vi "Ball Collector SM 5.1.vi"(1 "FIRE":bool, 2 "REVERSE":bool, 3 "Intake Motor":bool, 4 "OVERRIDE":bool, 5 "OVERRIDE 2":bool, 8 "BB1":bool, 9 "1":bool, 10 "BB2":bool, 11 "2":bool, 12 "BB3":bool, 13 "3":bool, 14 "BB4":bool, 27 "new behavior":bool) -> (20 "Ball Count":dbl, 21 "Intake motor":dbl, 22 "Motor A 2":dbl, 23 "Motor B 3":dbl, 24 "Motor C":dbl)   [LabVIEW 2011]
panel:
  in  "Feed Delay (sec) 2":dbl=0.5
  in  "Feed Delay (sec)":dbl=0.5
  in  "Prime":dbl(knob)=0.20200759564815568 scale=0.0..1.0
  in  "FIRE":dbl(knob)=0.5049245430258039 scale=0.0..1.0
  out "C from 3":bool
  out "B from 2":bool
  out "A from 1":bool
  out "BSB State":enum16{"Ball Entered"}(ring)
  out "BSC":bool
  out "BSB":bool
  out "BSA":bool
  out "MC":enum16{"Stopped", "Foward", "Reverse"}(ring)
  out "MA":enum16{"Stopped", "Foward", "Reverse"}(ring)
  out "MB":enum16{"Stopped", "Foward", "Reverse"}(ring)
  out "Intake motor":bool
  out "C Status":string
  out "B Status":string
  out "A Status":string
  out "Ball System State":string
  out "Primed":bool
  out "MA":bool
  out "MB":bool
  out "MC":bool
  # "Upper System"
  # "Upper/Middle System (U/M)"
  # "Ball systems"
  # "Vacant = Black (T)\nOccupied = Orange (F)"
  # "Lower/Middle System (L/M)"
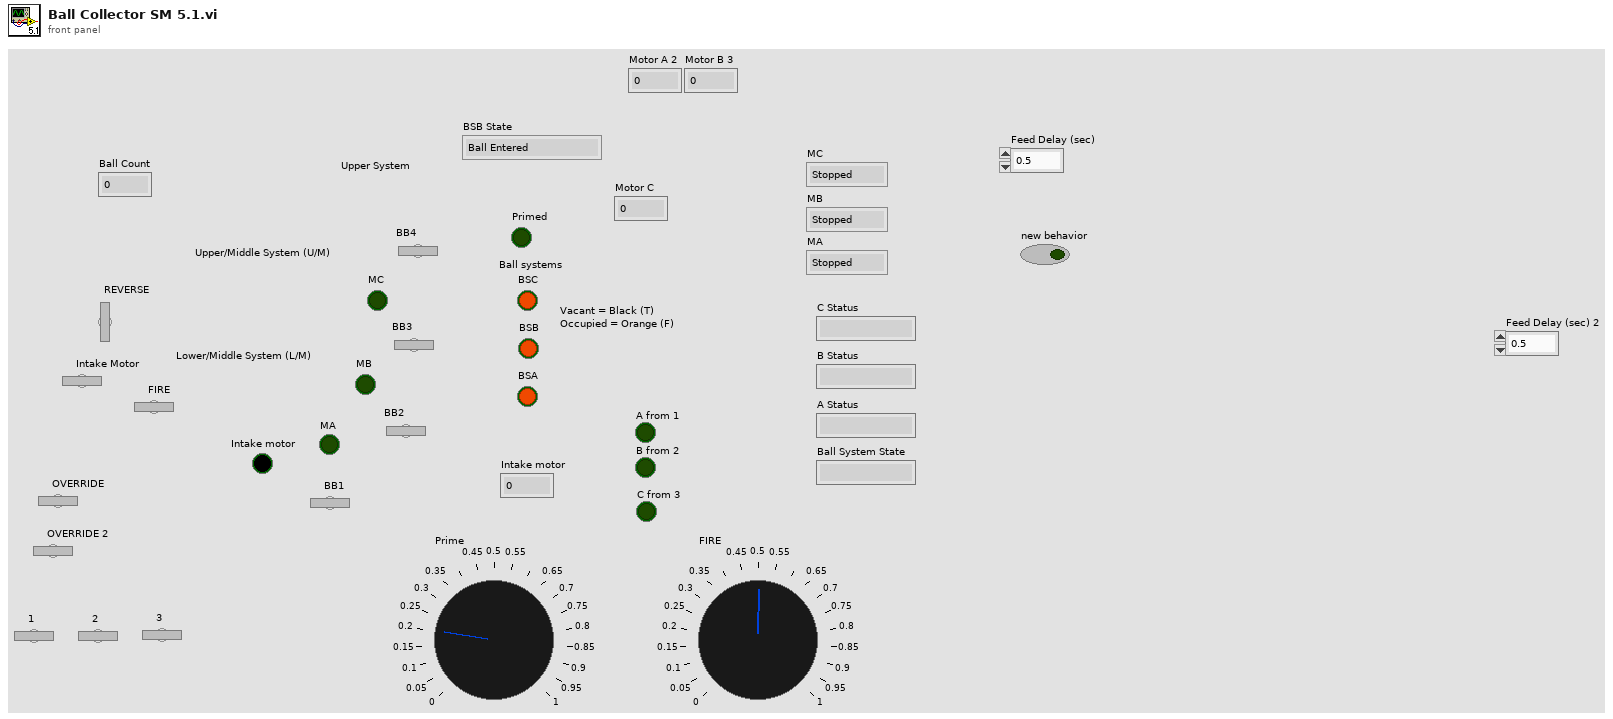
[diagram p1: front panel]
types:
  T1 = enum16{"Ball Entered", "Ball Stopped", "Ball Moveing", "Ball Leaving"}
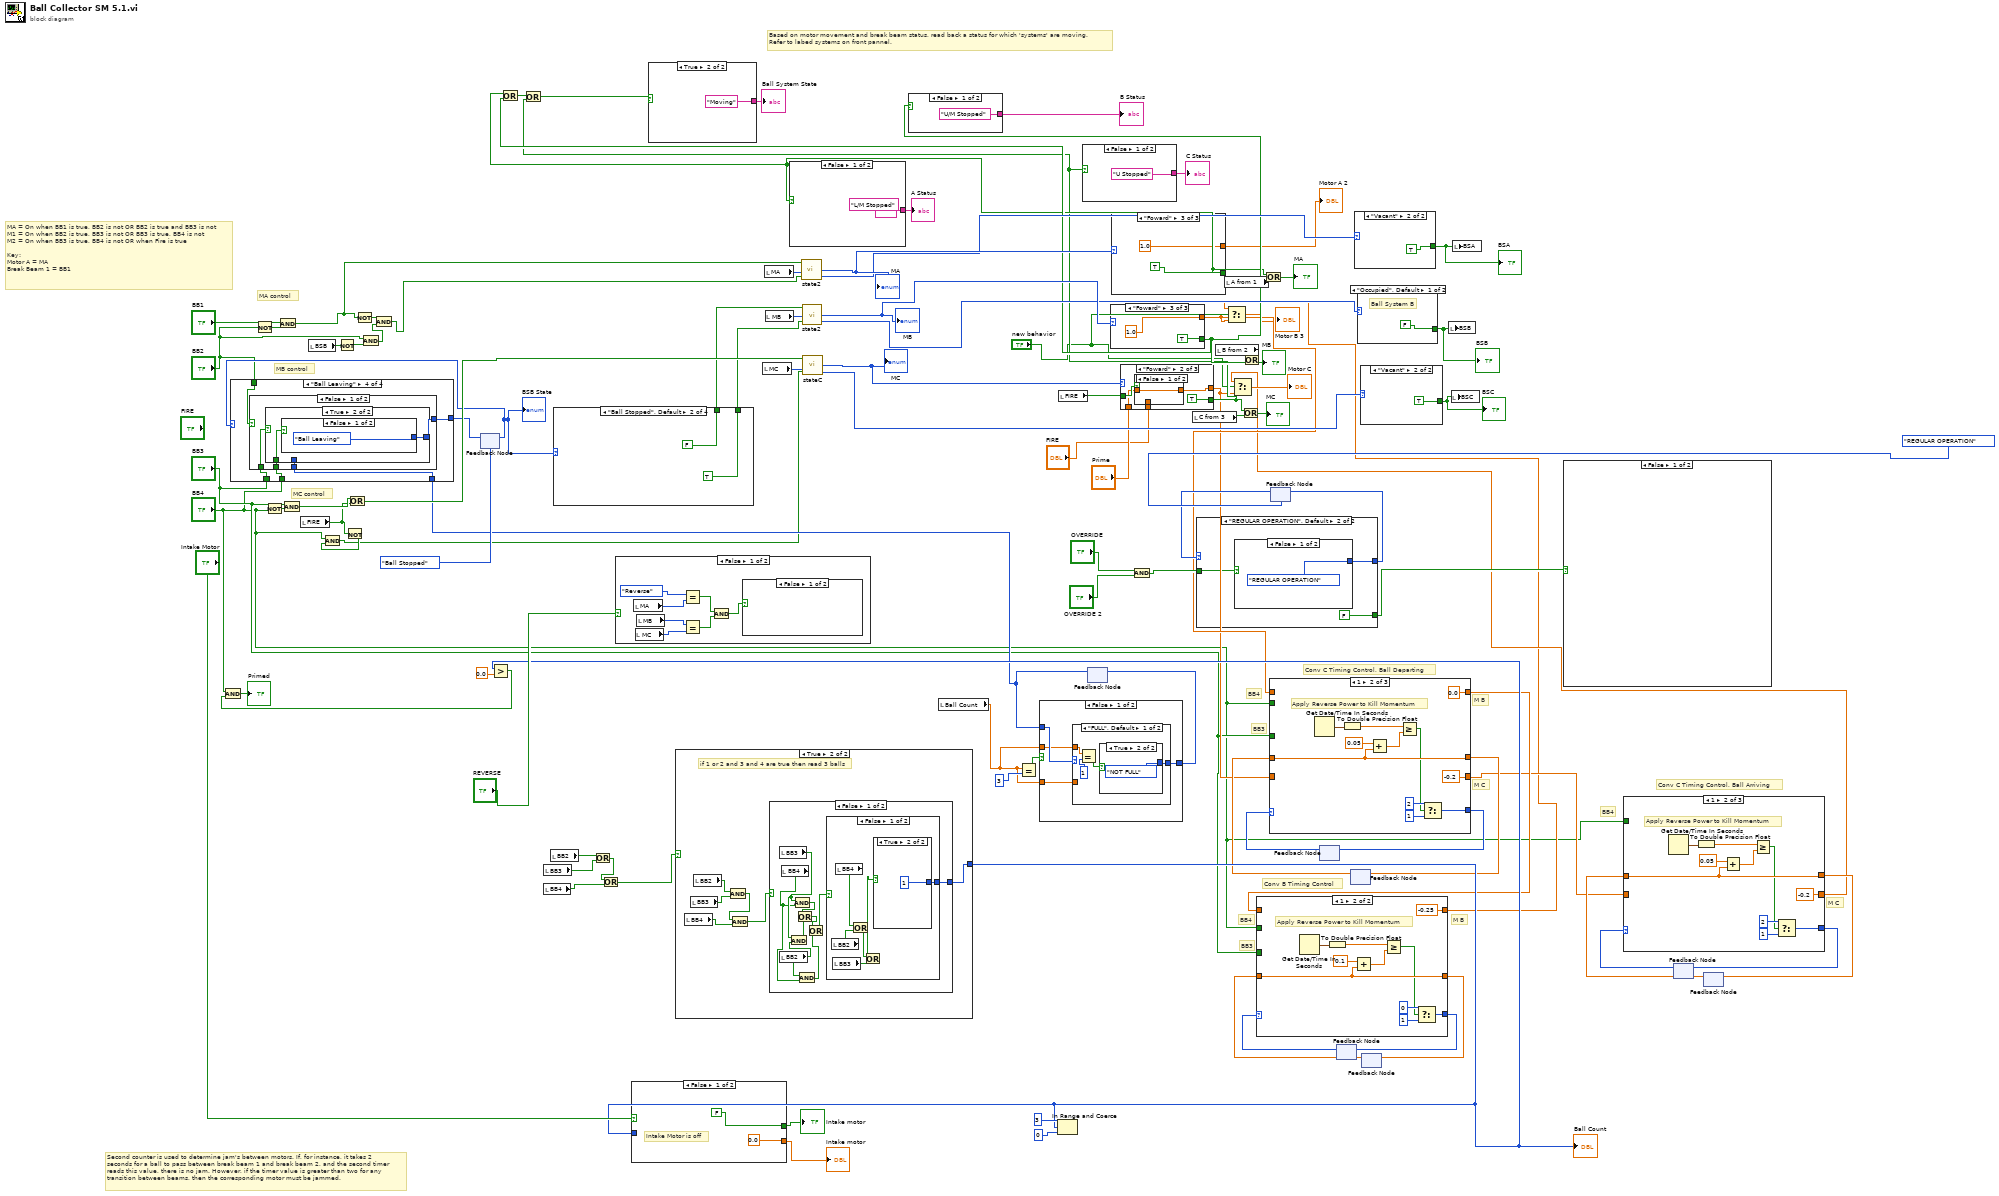
[diagram p0: block diagram]
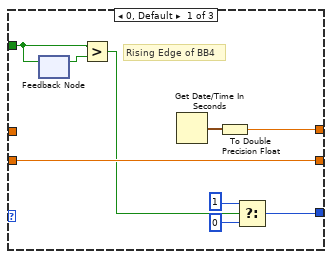
[diagram p2: hidden frame]
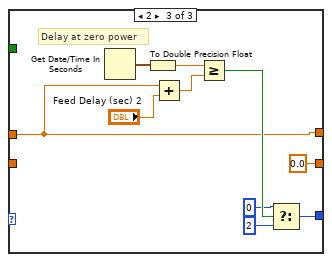
[diagram p3: hidden frame]
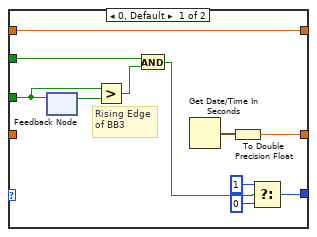
[diagram p4: hidden frame]
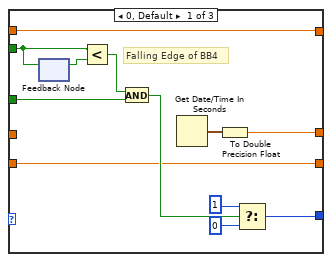
[diagram p5: hidden frame]
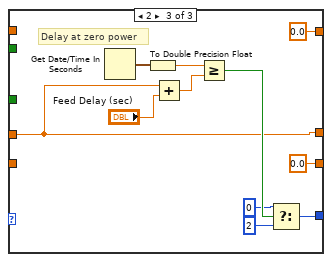
[diagram p6: hidden frame]
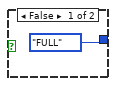
[diagram p7: hidden frame]
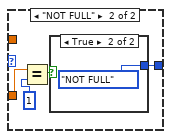
[diagram p8: hidden frame]
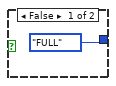
[diagram p9: hidden frame]
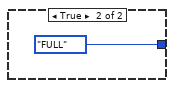
[diagram p10: hidden frame]
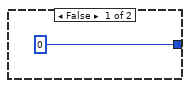
[diagram p11: hidden frame]
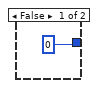
[diagram p12: hidden frame]
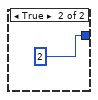
[diagram p13: hidden frame]
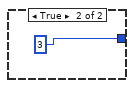
[diagram p14: hidden frame]
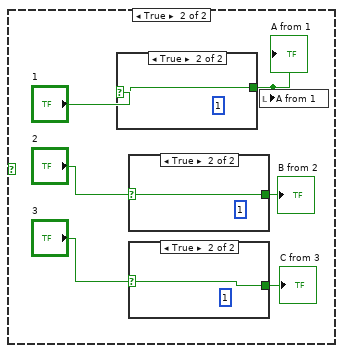
[diagram p15: hidden frame]
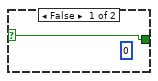
[diagram p16: hidden frame]
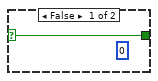
[diagram p17: hidden frame]
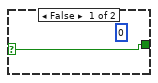
[diagram p18: hidden frame]
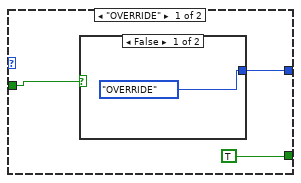
[diagram p19: hidden frame]
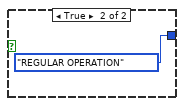
[diagram p20: hidden frame]
diagram:
  # "M C"
  # "BB4"
  # "Conv C Timing Control, Ball Arriving"
  # "Conv C Timing Control, Ball Departing"
  # "M B"
  # "M C"
  # "M B"
  # "BB4"
  # "BB3"
  # "BB3"
  # "BB4"
  # "Conv B Timing Control"
  # "MC control"
  # "MB control"
  # "MA control"
  # "Second counter is used to determine jam's between motors. If, for instance, it takes 2\nseconds for a ball to pass between break beam 1 and break beam 2, and the second timer\nreads this value, there is no jam. However, if the timer value is greater than two for any\ntransition between beams, then the corresponding motor must be jammed."
  # "Based on motor movement and break beam status, read back a status for which 'systems' are moving.\nRefer to labed systems on front pannel."
  # "MA = On when BB1 is true, BB2 is not OR BB2 is true and BB3 is not\nM1 = On when BB2 is true, BB3 is not OR BB3 is true, BB4 is not\nM2 = On when BB3 is true, BB4 is not OR when Fire is true\n\nKey:\nMotor A = MA\nBreak Beam 1 = BB1"
  n1 = Not(x="BB2") -> (.not. x?=w79:bool)
  n2 = Not(x="BB4") -> (.not. x?=w78:bool)
  n3 = And(x="BB1", y=w79) -> (x .and. y?=w66:bool)
  n4 = And(x="BB3", y=w78) -> (x .and. y?=w77:bool)
  n5 = local read "FIRE"() -> (w37:bool)
  n6 = local read "BSB"() -> (w76:bool)
  n7 = Not(x=w76) -> (.not. x?=w75:bool)
  n8 = Not(x=w37) -> (.not. x?=w27:bool)
  n9 = And(x="BB4", y=w27) -> (x .and. y?=w26:bool)
  n10 = Or(x=w77, y=w37) -> (x .or. y?=w67:bool)
  n11 = Not(x=w66) -> (.not. x?=w72:bool)
  n12 = And(x="BB2", y=w75) -> (x .and. y?=w74:bool)
  n13 = And(x=w72, y=w74) -> (x .and. y?=w73:bool)
  n14 = feedback #1(T1."Ball Stopped") -> (w58:T1)
  "BSB State" <- w58
  n15 = local read "BB4"() -> (w40:bool)
  n16 = local read "BB3"() -> (w39:bool)
  n17 = local read "BB2"() -> (w41:bool)
  n18 = case shown="\"Ball Stopped\", Default" w58 {
    tunnel: [TRUE FALSE TRUE TRUE] -> w61
    tunnel: [FALSE TRUE FALSE FALSE] -> w60
    frame "Ball Entered" {
      (unwired) 0.0
    }
    frame "Ball Stopped", Default {
    }
    frame "Ball Moveing" {
      (unwired) 0.0
    }
    frame "Ball Leaving" {
      n19 = Get Date/Time In Seconds() -> (seconds since 1Jan1904=w108:timestamp)
      n20 = To Double Precision Float(number=w108) -> ()  [unwired: 1 out]
    }
  }
  n21 = Or(x=w41, y=w39) -> (x .or. y?=w42:bool)
  n22 = Or(x=w42, y=w40) -> (x .or. y?=w38:bool)
  n23 = case shown="False" "REVERSE" {
    frame False {
      n24 = local read "MA"() -> (w116:enum16{"Stopped", "Foward", "Reverse"})
      n25 = local read "MC"() -> (w114:enum16{"Stopped", "Foward", "Reverse"})
      n26 = local read "MB"() -> (w115:enum16{"Stopped", "Foward", "Reverse"})
      n27 = Equal?(x=enum16{"Stopped", "Foward", "Reverse"}."Reverse" ("value"), y=w116) -> (x = y?=w112:bool)
      n28 = Equal?(x=w115, y=w114) -> (x = y?=w113:bool)
      n29 = And(x=w112, y=w113) -> (x .and. y?=w111:bool)
      n30 = case shown="False" w111 {
        frame False {
        }
        frame True {
          w118 = enum16{"Stopped", "Foward", "Reverse"}."Stopped" ("value")
          n31 = local write "MA"(w118) -> ()
          n32 = local write "MB"(w118) -> ()
          n33 = local write "MC"(w118) -> ()
        }
      }
    }
    frame True {
      w119 = enum16{"Stopped", "Foward", "Reverse"}."Reverse" ("MB")
      n34 = local write "MC"(w119) -> ()
      n35 = local write "MA"(w119) -> ()
      n36 = local write "MB"(w119) -> ()
    }
  }
  n37 = case shown="True" w38 {
    tunnel: [0 w122] -> w36
    frame False {
    }
    frame True {
      # "if 1 or 2 and 3 and 4 are true then read 3 balls"
      n38 = local read "BB4"() -> (w123:bool)
      n39 = local read "BB3"() -> (w124:bool)
      n40 = local read "BB2"() -> (w125:bool)
      n41 = And(x=w125, y=w124) -> (x .and. y?=w126:bool)
      n42 = And(x=w126, y=w123) -> (x .and. y?=w121:bool)
      n43 = case shown="False" w121 {
        tunnel: [w135 3] -> w122
        frame False {
          n44 = local read "BB3"() -> (w132:bool)
          n45 = local read "BB2"() -> (w131:bool)
          n46 = local read "BB4"() -> (w130:bool)
          n47 = And(x=w132, y=w131) -> (x .and. y?=w133:bool)
          n48 = And(x=w132, y=w130) -> (x .and. y?=w134:bool)
          n49 = Or(x=w134, y=w133) -> (x .or. y?=w129:bool)
          n50 = And(x=w131, y=w130) -> (x .and. y?=w127:bool)
          n51 = Or(x=w129, y=w127) -> (x .or. y?=w128:bool)
          n52 = case shown="False" w128 {
            tunnel: [w141 2] -> w135
            frame False {
              n53 = local read "BB2"() -> (w140:bool)
              n54 = local read "BB3"() -> (w138:bool)
              n55 = local read "BB4"() -> (w136:bool)
              n56 = Or(x=w136, y=w140) -> (x .or. y?=w139:bool)
              n57 = Or(x=w139, y=w138) -> (x .or. y?=w137:bool)
              n58 = case shown="True" w137 {
                tunnel: [0 1] -> w141
                frame False {
                }
                frame True {
                }
              }
            }
            frame True {
            }
          }
        }
        frame True {
        }
      }
    }
  }
  "Ball Count" <- w36
  n59 = Greater?(x=w36, y=0.0 ("f")) -> (0:w93:bool)
  n60 = And(x="BB4", y=w93) -> (x .and. y?=→"Primed":bool)
  n61 = case shown="False" "Intake Motor" {
    tunnel: [FALSE w150] -> w96
    tunnel: [0.0 w149] -> w70
    tunnel: w36 -> [_ w148]
    frame False {
      # "Intake Motor is off"
    }
    frame True {
      # "Only allow the intake\nmotor to be on if\nthere are less than\n3 Ballz"
      n62 = Less?(x=w148, y=3) -> (x < y?=w151:bool)
      n63 = case shown="False" w151 {
        selector: w151 -> [_ w156]
        tunnel: [TRUE w156] -> w150
        tunnel: [-1 1] -> w149
        frame False {
        }
        frame True {
        }
      }
    }
  }
  "Intake motor" <- w96
  "Intake motor" <- w70
  n64 = local read "MC"() -> (w89:enum16{"Stopped", "Foward", "Reverse"})
  n65 = local read "MA"() -> (w90:enum16{"Stopped", "Foward", "Reverse"})
  n66 = local read "MB"() -> (w91:enum16{"Stopped", "Foward", "Reverse"})
  n67 = call "state2.vi"("Stop/Transfer"=w73, "State"=w90, "Start"=w66) -> ("Ball State"=w83:enum16{"Occupied", "Vacant"}, "OutState"=w88:enum16{"Stopped", "Foward", "Reverse"})  [unwired: 1 in]
  "MA" <- w88
  n68 = call "state2.vi"("Stop/Transfer"=w60, "State"=w91, "Start"=w61) -> ("Ball State"=w84:enum16{"Occupied", "Vacant"}, "OutState"=w87:enum16{"Stopped", "Foward", "Reverse"})  [unwired: 1 in]
  "MB" <- w87
  n69 = call "stateC.vi"("Stop/Transfer"=w26, "State"=w89, "Start"=w67) -> ("Ball State"=w85:enum16{"Occupied", "Vacant"}, "OutState"=w86:enum16{"Stopped", "Foward", "Reverse"})  [unwired: 1 in]
  "MC" <- w86
  n70 = local read "Ball Count"() -> (w31:dbl)
  n71 = Equal?(x=w31, y=3) -> (x = y?=w34:bool)
  n72 = In Range and Coerce(upper limit=3, x=w36, lower limit=0) -> ()  [unwired: 2 out]
  n73 = local read "FIRE"() -> (w29:bool)
  n74 = feedback #2() -> (w32:enum16{"FULL", "NOT FULL"})  [unwired: 1 in]
  n75 = case shown="\"Ball Leaving\"" w58 {
    tunnel: "BB2" -> [w160 w180 w200 w223]
    tunnel: "BB3" -> [w159 w179 w199 w225]
    tunnel: "BB4" -> [w158 w178 w198 w224]
    tunnel: [w157 w177 w201 w226] -> w59
    tunnel: w32 -> [_ _ w197 w222]
    frame "Ball Entered" {
      n76 = case shown="False" w160 {
        tunnel: [w163 w171] -> w157
        tunnel: w159 -> [w162 w169]
        tunnel: w158 -> [w161 w170]
        frame False {
          n77 = case shown="False" w162 {
            tunnel: [T1."Ball Entered" w166] -> w163
            tunnel: w161 -> [_ w165]
            frame False {
            }
            frame True {
              n78 = case shown="False" w165 {
                tunnel: [T1."Ball Leaving" T1."Ball Stopped"] -> w166
                frame False {
                }
                frame True {
                }
              }
            }
          }
        }
        frame True {
          n79 = case shown="False" w169 {
            tunnel: [T1."Ball Entered" w174] -> w171
            tunnel: w170 -> [_ w173]
            frame False {
            }
            frame True {
              n80 = case shown="False" w173 {
                tunnel: [T1."Ball Leaving" T1."Ball Stopped"] -> w174
                frame False {
                }
                frame True {
                }
              }
            }
          }
        }
      }
    }
    frame "Ball Stopped", Default {
      n81 = case shown="True" w180 {
        tunnel: [w183 w191] -> w177
        tunnel: w179 -> [w182 w189]
        tunnel: w178 -> [w181 w190]
        frame False {
          n82 = case shown="False" w182 {
            tunnel: [T1."Ball Stopped" w186] -> w183
            tunnel: w181 -> [_ w185]
            frame False {
            }
            frame True {
              n83 = case shown="True" w185 {
                tunnel: [T1."Ball Leaving" T1."Ball Stopped"] -> w186
                frame False {
                }
                frame True {
                }
              }
            }
          }
        }
        frame True {
          n84 = case shown="True" w189 {
            tunnel: [T1."Ball Entered" w194] -> w191
            tunnel: w190 -> [_ w193]
            frame False {
            }
            frame True {
              n85 = case shown="False" w193 {
                tunnel: [T1."Ball Leaving" T1."Ball Stopped"] -> w194
                frame False {
                }
                frame True {
                }
              }
            }
          }
        }
      }
    }
    frame "Ball Moveing" {
      n86 = case shown="False" w200 {
        tunnel: [w205 w216] -> w201
        tunnel: w199 -> [w204 w214]
        tunnel: w198 -> [w203 w215]
        tunnel: w197 -> [w202 _]
        frame False {
          n87 = case shown="False" w204 {
            tunnel: [w207 w211] -> w205
            tunnel: w203 -> [_ w210]
            tunnel: w202 -> [w206 _]
            frame False {
              n88 = case shown="\"NOT FULL\"" w206 {
                tunnel: [T1."Ball Moveing" T1."Ball Stopped"] -> w207
                frame "FULL", Default {
                }
                frame "NOT FULL" {
                }
              }
            }
            frame True {
              n89 = case shown="True" w210 {
                tunnel: [T1."Ball Moveing" T1."Ball Stopped"] -> w211
                frame False {
                }
                frame True {
                }
              }
            }
          }
        }
        frame True {
          n90 = case shown="False" w214 {
            tunnel: [T1."Ball Entered" w219] -> w216
            tunnel: w215 -> [_ w218]
            frame False {
            }
            frame True {
              n91 = case shown="False" w218 {
                tunnel: [T1."Ball Leaving" T1."Ball Stopped"] -> w219
                frame False {
                }
                frame True {
                }
              }
            }
          }
        }
      }
    }
    frame "Ball Leaving" {
      n92 = case shown="False" w223 {
        tunnel: [w227 w241] -> w226
        tunnel: w225 -> [w230 w239]
        tunnel: w224 -> [w229 w240]
        tunnel: w222 -> [w228 _]
        frame False {
          n93 = case shown="True" w230 {
            tunnel: [w232 w236] -> w227
            tunnel: w229 -> [_ w235]
            tunnel: w228 -> [w231 _]
            frame False {
              n94 = case shown="\"NOT FULL\"" w231 {
                tunnel: [T1."Ball Moveing" T1."Ball Stopped"] -> w232
                frame "FULL", Default {
                }
                frame "NOT FULL" {
                }
              }
            }
            frame True {
              n95 = case shown="False" w235 {
                tunnel: [T1."Ball Leaving" T1."Ball Stopped"] -> w236
                frame False {
                }
                frame True {
                }
              }
            }
          }
        }
        frame True {
          n96 = case shown="True" w239 {
            tunnel: [T1."Ball Entered" w244] -> w241
            tunnel: w240 -> [_ w243]
            frame False {
            }
            frame True {
              n97 = case shown="False" w243 {
                tunnel: [T1."Ball Leaving" T1."Ball Stopped"] -> w244
                frame False {
                }
                frame True {
                }
              }
            }
          }
        }
      }
    }
  }
  n98 = feedback-in #1(w59) -> ()
  n99 = case shown="False" w34 {
    tunnel: w32 -> [w250 _]
    tunnel: [w249 enum16{"FULL", "NOT FULL"}."FULL"] -> w33
    tunnel: w31 -> [w248 _]
    tunnel: w31 -> [w247 _]
    frame False {
      n100 = case shown="\"FULL\", Default" w250 {
        tunnel: [w251 w260] -> w249
        tunnel: w248 -> [_ w259]
        tunnel: w247 -> [w252 _]
        frame "FULL", Default {
          n101 = Equal?(x=w252, y=1) -> (x = y?=w254:bool)
          n102 = case shown="True" w254 {
            tunnel: [enum16{"FULL", "NOT FULL"}."FULL" enum16{"FULL", "NOT FULL"}."NOT FULL"] -> w251
            frame False {
            }
            frame True {
            }
          }
        }
        frame "NOT FULL" {
          n103 = Equal?(x=w259, y=1) -> (x = y?=w258:bool)
          n104 = case shown="True" w258 {
            tunnel: [enum16{"FULL", "NOT FULL"}."FULL" enum16{"FULL", "NOT FULL"}."NOT FULL"] -> w260
            frame False {
            }
            frame True {
            }
          }
        }
      }
    }
    frame True {
    }
  }
  n105 = feedback-in #2(w33) -> ()
  n106 = case shown="\"Foward\"" w87 {
    tunnel: [FALSE TRUE TRUE] -> w65
    tunnel: [0.0 -1.0 1.0] -> w20
    frame "Stopped", Default {
    }
    frame "Reverse" {
    }
    frame "Foward" {
    }
  }
  n107 = case shown="False" w65 {
    tunnel: ["U/M Stopped" "U/M Moving"] -> w98
    frame False {
    }
    frame True {
    }
  }
  "B Status" <- w98
  n108 = case shown="\"Foward\"" w88 {
    tunnel: [FALSE TRUE TRUE] -> w56
    tunnel: [0.0 -1.0 1.0] -> w25
    frame "Stopped", Default {
    }
    frame "Reverse" {
    }
    frame "Foward" {
    }
  }
  "Motor A 2" <- w25
  n109 = Or(x=w56, y=w65) -> (x .or. y?=w69:bool)
  n110 = case shown="False" w56 {
    tunnel: ["L/M Stopped" "L/M Moving up"] -> w99
    frame False {
    }
    frame True {
    }
  }
  "A Status" <- w99
  n111 = case shown="\"Foward\"" w86 {
    tunnel: [0.0 w284 -1.0] -> w17
    tunnel: [FALSE TRUE TRUE] -> w50
    tunnel: "Prime" -> [_ w282 _]
    tunnel: w29 -> [_ w285 _]
    tunnel: "FIRE" -> [_ w283 _]
    frame "Stopped", Default {
    }
    frame "Foward" {
      n112 = case shown="False" w285 {
        tunnel: [w287 w288] -> w284
        tunnel: w283 -> [_ w288]
        tunnel: w282 -> [w287 _]
        frame False {
        }
        frame True {
        }
      }
    }
    frame "Reverse" {
    }
  }
  n113 = Or(x=w69, y=w50) -> (x .or. y?=w68:bool)
  n114 = case shown="True" w68 {
    tunnel: ["Stopped" "Moving"] -> w100
    frame False {
    }
    frame True {
    }
  }
  "Ball System State" <- w100
  n115 = case shown="False" w50 {
    tunnel: ["U Stopped" "Firing"] -> w97
    frame False {
    }
    frame True {
    }
  }
  "C Status" <- w97
  n116 = And(x="OVERRIDE", y="OVERRIDE 2") -> (x .and. y?=w46:bool)
  n117 = local read "C from 3"() -> (w49:bool)
  n118 = local read "B from 2"() -> (w52:bool)
  n119 = local read "A from 1"() -> (w53:bool)
  n120 = Or(x=w50, y=w49) -> (x .or. y?=→"MC":bool)
  n121 = Or(x=w52, y=w65) -> (x .or. y?=→"MB":bool)
  n122 = Or(x=w56, y=w53) -> (x .or. y?=→"MA":bool)
  n123 = feedback #3(enum16{"OVERRIDE", "REGULAR OPERATION"}."REGULAR OPERATION") -> (w47:enum16{"OVERRIDE", "REGULAR OPERATION"})
  n124 = case shown="\"REGULAR OPERATION\", Default" w47 {
    tunnel: [w296 w302] -> w48
    tunnel: w46 -> [w297 w301]
    tunnel: [TRUE FALSE] -> w45
    frame "OVERRIDE" {
      n125 = case shown="False" w297 {
        tunnel: [enum16{"OVERRIDE", "REGULAR OPERATION"}."OVERRIDE" enum16{"OVERRIDE", "REGULAR OPERATION"}."REGULAR OPERATION"] -> w296
        frame False {
        }
        frame True {
        }
      }
    }
    frame "REGULAR OPERATION", Default {
      n126 = case shown="False" w301 {
        tunnel: [enum16{"OVERRIDE", "REGULAR OPERATION"}."REGULAR OPERATION" enum16{"OVERRIDE", "REGULAR OPERATION"}."OVERRIDE"] -> w302
        frame False {
        }
        frame True {
        }
      }
    }
  }
  n127 = feedback-in #3(w48) -> ()
  n128 = feedback #4() -> (w23:i64)  [unwired: 1 in]
  n129 = feedback #5() -> (w15:i64)  [unwired: 1 in]
  n130 = feedback #6() -> (w21:dbl)  [unwired: 1 in]
  n131 = case shown="1" w23 {
    tunnel: [w314 w323 w328] -> w24
    tunnel: "BB4" -> [w315 _ _]
    tunnel: "BB3" -> [w310 _ _]
    tunnel: w17 -> [w308 _ _]
    tunnel: [w308 -0.2 ("FIRE") 0.0 ("FIRE")] -> w6
    tunnel: [w306 w321 w331] -> w22
    tunnel: w21 -> [_ w321 w331]
    tunnel: w20 -> [w305 _ _]
    tunnel: [w305 0.0 0.0] -> w12
    frame 0, Default {
      # "Falling Edge of BB4"
      n132 = feedback-in #7(w315) -> ()
      n133 = feedback #7() -> (w316:bool)  [unwired: 1 in]
      n134 = Less?(x=w315, y=w316) -> (x < y?=w311:bool)
      n135 = And(x=w311, y=w310) -> (x .and. y?=w309:bool)
      n136 = Get Date/Time In Seconds() -> (seconds since 1Jan1904=w307:timestamp)
      n137 = To Double Precision Float(number=w307) -> (double precision float=w306:dbl)
      n138 = Select(t=1, s=w309, f=0) -> (s? t:f=w314:i32)
    }
    frame 1 {
      # "Apply Reverse Power to Kill Momentum"
      n139 = Get Date/Time In Seconds() -> (seconds since 1Jan1904=w327:timestamp)
      n140 = To Double Precision Float(number=w327) -> (double precision float=w319:dbl)
      n141 = Add(x=0.05, y=w321) -> (x+y=w318:dbl)
      n142 = Greater Or Equal?(x=w319, y=w318) -> (x >= y?=w317:bool)
      n143 = Select(t=i64 2, s=w317, f=i64 1) -> (s? t:f=w323:i64)
    }
    frame 2 {
      # "Delay at zero power"
      n144 = Get Date/Time In Seconds() -> (seconds since 1Jan1904=w337:timestamp)
      n145 = To Double Precision Float(number=w337) -> (double precision float=w336:dbl)
      n146 = Add(x=w331, y="Feed Delay (sec)") -> (x+y=w335:dbl)
      n147 = Greater Or Equal?(x=w336, y=w335) -> (x >= y?=w334:bool)
      n148 = Select(t=0, s=w334, f=2) -> (s? t:f=w328:i32)
    }
  }
  n149 = feedback-in #4(w24) -> ()
  n150 = feedback-in #6(w22) -> ()
  n151 = case shown="\"Vacant\"" w83 {
    tunnel: [FALSE TRUE] -> w81
    frame "Occupied", Default {
      # "Ball System A"
    }
    frame "Vacant" {
    }
  }
  "BSA" <- w81
  n152 = case shown="\"Occupied\", Default" w84 {
    tunnel: [FALSE TRUE] -> w82
    frame "Occupied", Default {
      # "Ball System B"
    }
    frame "Vacant" {
    }
  }
  "BSB" <- w82
  n153 = case shown="\"Vacant\"" w85 {
    tunnel: [FALSE TRUE] -> w80
    frame "Occupied", Default {
      # "Ball System C"
    }
    frame "Vacant" {
    }
  }
  "BSC" <- w80
  n154 = feedback #8() -> (w13:dbl)  [unwired: 1 in]
  n155 = case shown="1" w15 {
    tunnel: "BB4" -> [w347 _]
    tunnel: "BB3" -> [w349 _]
    tunnel: [w355 w359] -> w16
    tunnel: [w351 w358] -> w14
    tunnel: w13 -> [_ w358]
    tunnel: w12 -> [w345 _]
    tunnel: [w345 -0.25] -> w4
    frame 0, Default {
      # "Rising Edge\nof BB3"
      n156 = feedback-in #9(w349) -> ()
      n157 = feedback #9() -> (w350:bool)  [unwired: 1 in]
      n158 = Greater?(x=w349, y=w350) -> (0:w348:bool)
      n159 = And(x=w347, y=w348) -> (x .and. y?=w346:bool)
      n160 = Get Date/Time In Seconds() -> (seconds since 1Jan1904=w352:timestamp)
      n161 = To Double Precision Float(number=w352) -> (double precision float=w351:dbl)
      n162 = Select(t=1, s=w346, f=0) -> (s? t:f=w355:i32)
    }
    frame 1 {
      # "Apply Reverse Power to Kill Momentum"
      n163 = Get Date/Time In Seconds() -> (seconds since 1Jan1904=w362:timestamp)
      n164 = To Double Precision Float(number=w362) -> (double precision float=w364:dbl)
      n165 = Add(x=0.1, y=w358) -> (x+y=w365:dbl)
      n166 = Greater Or Equal?(x=w364, y=w365) -> (x >= y?=w356:bool)
      n167 = Select(t=i64 0, s=w356, f=i64 1) -> (s? t:f=w359:i64)
    }
  }
  n168 = Select(t=w4, s="new behavior", f=w20) -> (s? t:f=→"Motor B 3":dbl)
  n169 = feedback-in #5(w16) -> ()
  n170 = feedback-in #8(w14) -> ()
  n171 = local write "BSB"(w82) -> ()
  n172 = local write "BSC"(w80) -> ()
  n173 = local write "BSA"(w81) -> ()
  n174 = case shown="False" w45 {
    frame False {
    }
    frame True {
      n175 = case shown="True" "1" {
        selector: "1" -> [w376 w377]
        tunnel: [w376 w377] -> w368
        frame False {
          (unwired) 0
        }
        frame True {
          (unwired) 1
        }
      }
      "A from 1" <- w368
      n176 = case shown="True" "2" {
        selector: "2" -> [w374 w375]
        tunnel: [w374 w375] -> w366
        frame False {
          (unwired) 0
        }
        frame True {
          (unwired) 1
        }
      }
      "B from 2" <- w366
      n177 = case shown="True" "3" {
        selector: "3" -> [w372 w373]
        tunnel: [w372 w373] -> w367
        frame False {
          (unwired) 0
        }
        frame True {
          (unwired) 1
        }
      }
      "C from 3" <- w367
      n178 = local write "A from 1"(w368) -> ()
    }
  }
  n179 = feedback #10() -> (w9:i64)  [unwired: 1 in]
  n180 = feedback #11() -> (w11:dbl)  [unwired: 1 in]
  n181 = case shown="1" w9 {
    tunnel: [w384 w393 w397] -> w8
    tunnel: "BB4" -> [w385 _ _]
    tunnel: w6 -> [w381 _ _]
    tunnel: [w381 -0.2 ("FIRE") 0.0 ("FIRE")] -> w5
    tunnel: [w379 w391 w399] -> w10
    tunnel: w11 -> [_ w391 w399]
    frame 0, Default {
      # "Rising Edge of BB4"
      n182 = feedback-in #12(w385) -> ()
      n183 = feedback #12() -> (w386:bool)  [unwired: 1 in]
      n184 = Greater?(x=w385, y=w386) -> (0:w378:bool)
      n185 = Get Date/Time In Seconds() -> (seconds since 1Jan1904=w380:timestamp)
      n186 = To Double Precision Float(number=w380) -> (double precision float=w379:dbl)
      n187 = Select(t=1, s=w378, f=0) -> (s? t:f=w384:i32)
    }
    frame 1 {
      # "Apply Reverse Power to Kill Momentum"
      n188 = Get Date/Time In Seconds() -> (seconds since 1Jan1904=w396:timestamp)
      n189 = To Double Precision Float(number=w396) -> (double precision float=w389:dbl)
      n190 = Add(x=0.05, y=w391) -> (x+y=w388:dbl)
      n191 = Greater Or Equal?(x=w389, y=w388) -> (x >= y?=w387:bool)
      n192 = Select(t=i64 2, s=w387, f=i64 1) -> (s? t:f=w393:i64)
    }
    frame 2 {
      # "Delay at zero power"
      n193 = Get Date/Time In Seconds() -> (seconds since 1Jan1904=w405:timestamp)
      n194 = To Double Precision Float(number=w405) -> (double precision float=w404:dbl)
      n195 = Add(x=w399, y="Feed Delay (sec) 2") -> (x+y=w403:dbl)
      n196 = Greater Or Equal?(x=w404, y=w403) -> (x >= y?=w402:bool)
      n197 = Select(t=0, s=w402, f=2) -> (s? t:f=w397:i32)
    }
  }
  n198 = Select(t=w5, s="new behavior", f=w17) -> (s? t:f=→"Motor C":dbl)
  n199 = feedback-in #10(w8) -> ()
  n200 = feedback-in #11(w10) -> ()
